vi "Microscope.StopDependencies.vi"(8 "error in (no error)":errorcluster, 11 "Microscope in":refnum<class "Microscope.lvclass">) -> (0 "error out":errorcluster, 3 "Microscope out":refnum<class "Microscope.lvclass">)   [LabVIEW 2013, in "Microscope.lvclass"]
uses:
  Microscope.lvclass
  <vilib>/JKI/JKI SMO/SMO/SMO.lvclass
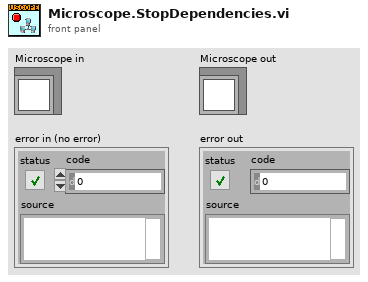
[diagram p1: front panel]
types:
  T1 = typedef "Microscope.lvclass/Dependencies--Cluster.ctl" = cluster{"XYStage":refnum<class "XYStage.lvclass">, "Camera":refnum<class "Camera.lvclass">}
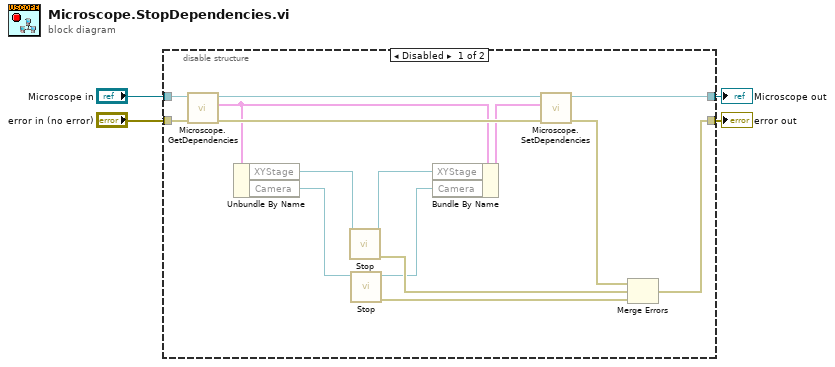
[diagram p0: block diagram]
diagram:
  n1 = disable-structure shown="Disabled" {
    disable-tunnel: "error in (no error)" -> [w19 w20]
    disable-tunnel: "Microscope in" -> [w18 w21]
    disable-tunnel: [w16 w21] -> w2
    disable-tunnel: [w13 w20] -> w1
    frame Disabled {
      n2 = call "Microscope.GetDependencies.vi"("error in (no error)"=w19, "Microscope"=w18) -> ("error out"=w15:errorcluster, "Dependencies"=w11:T1, "Microscope out"=w17:refnum<class "Microscope.lvclass">)  [unwired: 7 in]
      n3 = Unbundle By Name(w11) -> ("XYStage"=w10:refnum<class "XYStage.lvclass">, "Camera"=w7:refnum<class "Camera.lvclass">)
      n4 = call <vilib>:"Stop.vi"("SMO"=w10) -> ("error out"=w8:errorcluster, "SMO out"=w9:refnum<class "XYStage.lvclass">)  [unwired: 9 in]
      n5 = call <vilib>:"Stop.vi"("SMO"=w7) -> ("error out"=w5:errorcluster, "SMO out"=w6:refnum<class "Camera.lvclass">)  [unwired: 9 in]
      n6 = Bundle By Name(cluster=w11, "XYStage"=w9, "Camera"=w6) -> (w12:T1)
      n7 = call "Microscope.SetDependencies.vi"("error in (no error)"=w15, "Dependencies"=w12, "Microscope"=w17) -> ("error out"=w14:errorcluster, "Microscope out"=w16:refnum<class "Microscope.lvclass">)  [unwired: 7 in]
      n8 = Merge Errors(w14, w8, w5) -> (w13:errorcluster)
    }
    frame Enabled {
    }
  }
  "error out" <- w1
  "Microscope out" <- w2
